vi "read_dynamixels_and_update.vi"(6 "Motors Enabled":bool[](array[boolean])=[TRUE, TRUE, TRUE], 7 "Motors IDs Found":u8[](array[numeric]), 8 "error in (no error)":errorcluster, 9 "Last read positions":dbl[](array[numeric]), 10 "Dynamixel Cycle Constant":T1, 11 "VISA Refnum in":refnum<visa-resource-name>) -> (0 "error out":errorcluster[](array[cluster]), 1 "Latest read positions (dyn)":dbl[](array[numeric]), 2 "Updated Dynamixle Cycles":T1, 3 "VISA Refnum out":refnum<visa-resource-name>, 5 "Dynamixel\nPositions (deg)":dbl[](array[numeric]))   [LabVIEW 2013]
uses:
  Data/TypeDefs/DynamixelCycleTracker.ctl
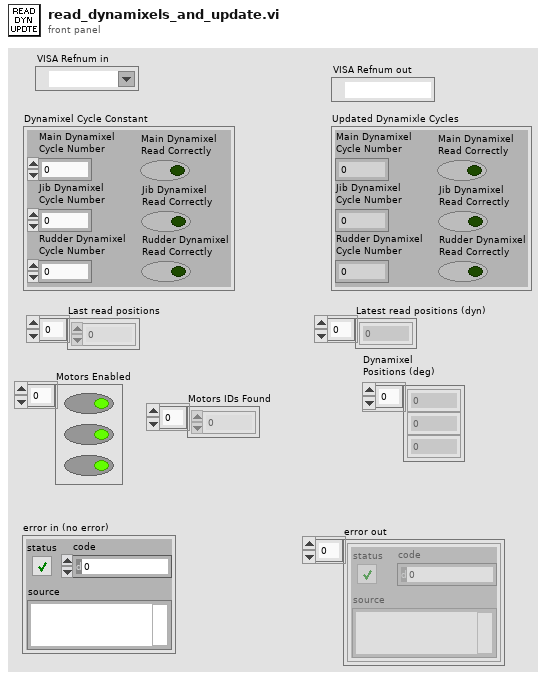
[diagram p1: front panel]
types:
  T1 = typedef "DynamixelCycleTracker.ctl" = cluster{"Main Dynamixel\nCycle Number":i32, "Jib Dynamixel\nCycle Number":i32, "Rudder Dynamixel\nCycle Number":i32, "Main Dynamixel\nRead Correctly":bool, "Jib Dynamixel\nRead Correctly":bool, "Rudder Dynamixel\nRead Correctly":bool}
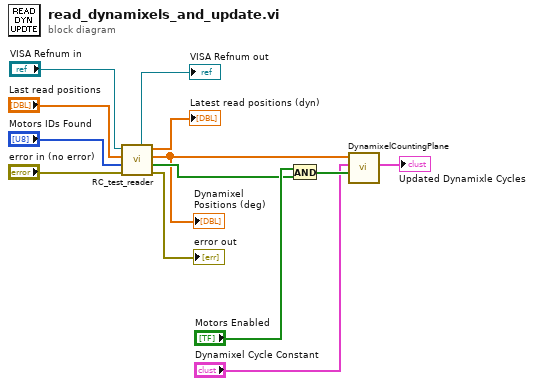
[diagram p0: block diagram]
diagram:
  n1 = call "RC_test_reader.vi"("error in (no error)"="error in (no error)", "Motors IDs Found"="Motors IDs Found", "Read positions (dyn)"="Last read positions", "VISA Refnum in"="VISA Refnum in") -> ("error out"=→"error out":errorcluster[], "Motors Read Correctly"=w10:bool[], "Dynamixel Positions (deg)"=w4:dbl[], "Read positions latest (dyn)"=→"Latest read positions (dyn)":dbl[], "VISA Refnum OUT"=→"VISA Refnum out":refnum<visa-resource-name>)  [unwired: 3 in]
  "Dynamixel\nPositions (deg)" <- w4
  n2 = And(x="Motors Enabled", y=w10) -> (x .and. y?=w9:bool[])
  n3 = call "DynamixelCountingPlane.vi"("Motors Read Correctly"=w9, "Dynamixel Cycles"="Dynamixel Cycle Constant", "Dynamixel Read Positions"=w4) -> ("Updated Dynamixle Cycles"=→"Updated Dynamixle Cycles":T1)  [unwired: 8 in]
